vi "Priority Dequeue.vi"(8 "error in (no error)":errorcluster, 9 "timeout in ms (-1)":i32=-1, 11 "Bounded Priority Queue in":refnum<class "Bounded Priority Queue.lvclass">) -> (0 "error out":errorcluster, 1 "timed out?":bool, 2 "element":T1, 3 "Bounded Priority Queue out":refnum<class "Bounded Priority Queue.lvclass">)   [LabVIEW 2011, in "Bounded Priority Queue.lvclass"]
uses:
  Bounded Priority Queue.lvclass
  Data.ctl
  Bounded Priority Queue.lvclass/Bounded Priority Queue.ctl
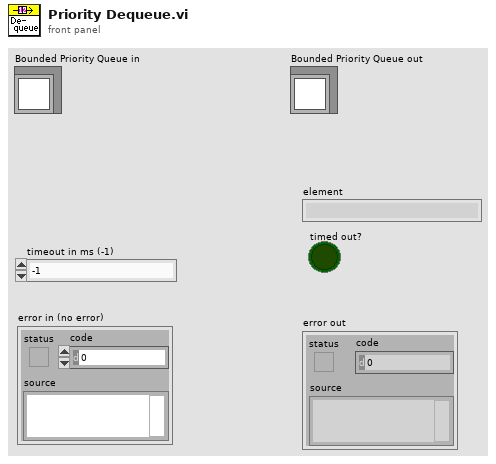
[diagram p1: front panel]
types:
  T1 = typedef "Bounded Priority Queue.lvclass/Data.ctl" = string
  T2 = typedef "Priority Queue.lvclass/DVR Contents.ctl" = cluster{"# Waiting":u32, "Buffers":refnum<queue>[], "How Many Priorities":u32, "Bounding":refnum<queue>}
  T3 = typedef "Priority Queue.lvclass/Data.ctl" = string
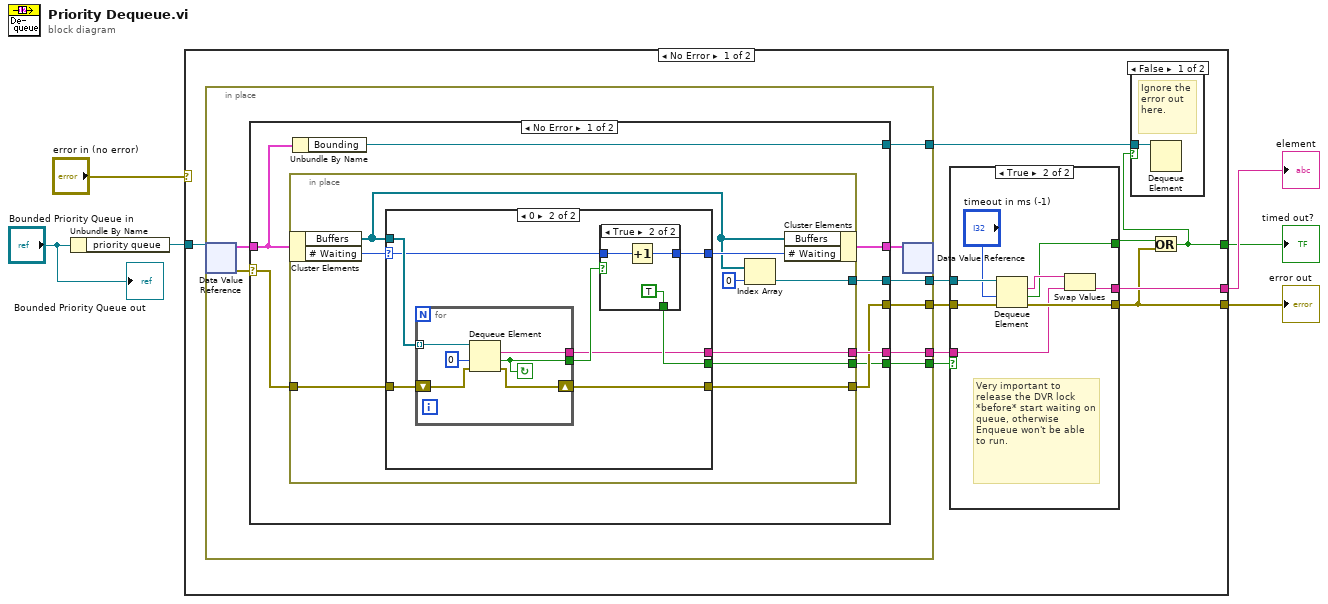
[diagram p0: block diagram]
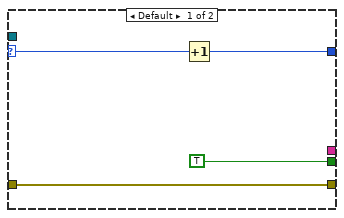
[diagram p4: hidden frame]
diagram:
  n1 = Unbundle By Name("Bounded Priority Queue in") -> ("priority queue"=w5:refnum<data-value>)
  n2 = case shown="No Error" "error in (no error)" {
    selector: "error in (no error)" -> [_ w77]
    tunnel: [w8 w77] -> w2
    tunnel: w5 -> [w16 _]
    tunnel: [w15 _] -> w3
    tunnel: [w7 _] -> w1
    frame No Error {
      n3 = in-place {
        in-place-border: [w34] -> w13
        in-place-border: [w31] -> w14
        in-place-border: [w30] -> w12
        in-place-border: [w29] -> w11
        in-place-border: [w28] -> w10
        n4 = in-place-dvr #1(w16) -> (w32:T2, w35:errorcluster)
        n5 = case shown="No Error" w35 {
          selector: w35 -> [w41 w76]
          tunnel: [w40 w76] -> w34
          tunnel: [w43 w75] -> w33
          tunnel: w32 -> [w37 w75]
          tunnel: [w42 _] -> w31
          tunnel: [w39 _] -> w30
          tunnel: [w38 _] -> w29
          tunnel: [w36 _] -> w28
          frame No Error {
            n6 = in-place {
              in-place-border: [w52] -> w42
              in-place-border: w41 -> [w49]
              in-place-border: [w48] -> w40
              in-place-border: [w47] -> w39
              in-place-border: [w45] -> w38
              n7 = in-place-cluster #2(w37) -> ("Buffers"=w44:refnum<queue>[], "# Waiting"=w51:u32)
              n8 = case shown="0" w51 {
                selector: w51 -> [w56 w62]
                tunnel: w44 -> [_ w64]
                tunnel: [_ w57] -> w52
                tunnel: [w55 w61] -> w50
                tunnel: w49 -> [w54 w60]
                tunnel: [w54 w59] -> w48
                tunnel: [TRUE w58] -> w47
                frame Default {
                  n9 = Increment(x=w56) -> (x+1=w55:u32)
                }
                frame 0 {
                  n10 = for {
                    tunnel: w64 -> [w69] mode=indexing
                    tunnel: [w73] -> w63
                    shift-right: [w71] -> w59
                    shift-left: w60 -> [w72]
                    tunnel: [w70] -> w57
                    stop <- w73 continue-if-true
                    n11 = Dequeue Element(queue=w69, timeout in ms (-1)=0, error in (no error)=w72) -> (element=w70:T3, timed out?=w73:bool, error out=w71:errorcluster)  [unwired: 1 out]
                  }
                  n12 = case shown="True" w63 {
                    tunnel: w62 -> [w65 w68]
                    tunnel: [w65 w67] -> w61
                    tunnel: [_ TRUE] -> w58
                    frame False {
                    }
                    frame True {
                      n13 = Increment(x=w68) -> (x+1=w67:u32)
                    }
                  }
                }
              }
              n14 = Index Array(array=w44, index=0) -> (element=w45:refnum<queue>)
              n15 = in-place-cluster #2("Buffers"=w44, "# Waiting"=w50) -> (w43:T2)
            }
            n16 = Unbundle By Name(w37) -> ("Bounding"=w36:refnum<queue>)
          }
          frame Error {
          }
        }
        n17 = in-place-dvr #1(w33) -> ()  [unwired: 2 out]
      }
      n18 = case shown="True" w12 {
        tunnel: [w19 w23] -> w15
        tunnel: w14 -> [w19 w22]
        tunnel: w13 -> [w18 w27]
        tunnel: [w18 w25] -> w8
        tunnel: w11 -> [_ w26]
        tunnel: [_ w20] -> w9
        frame False {
        }
        frame True {
          # "Very important to release the DVR lock *before* start waiting on queue, otherwise Enqueue won't be able to run."
          n19 = Dequeue Element(queue=w26, timeout in ms (-1)="timeout in ms (-1)", error in (no error)=w27) -> (element=w24:T3, timed out?=w20:bool, error out=w25:errorcluster)  [unwired: 1 out]
          n20 = Swap Values(12:w24, 14:w22) -> (3:w23:T3)  [unwired: 1 in, 1 out]
        }
      }
      n21 = Or(x=w9, y=w8) -> (x .or. y?=w7:bool)
      n22 = case shown="False" w7 {
        tunnel: w10 -> [w17 _]
        frame False {
          # "Ignore the error out here."
          n23 = Dequeue Element(queue=w17) -> ()  [unwired: 2 in, 4 out]
        }
        frame True {
        }
      }
    }
    frame Error {
    }
  }
  "element" <- w3
  "error out" <- w2
  "timed out?" <- w1
  "Bounded Priority Queue out" <- "Bounded Priority Queue in"
